vi "Delete_Unprocessed_Subtracks-1.vi"(4 "error IN":errorcluster, 5 "[IN] Before Pro\ncessing Tracks":T1(array[cluster]), 7 "[IN] Processed Tracks":T1(array[cluster])) -> (0 "error OUT":errorcluster, 1 "[OUT] Before Pro\ncessing Tracks":T1(array[cluster]), 3 "[IN] Filtered Tracks":T1(array[cluster]))   [LabVIEW 2013]
doc: "The subVI deletes the unprocessed points and tracks"
panel:
  out "# of deleted subtracks":i32
  out "# of deleted track groups":i32
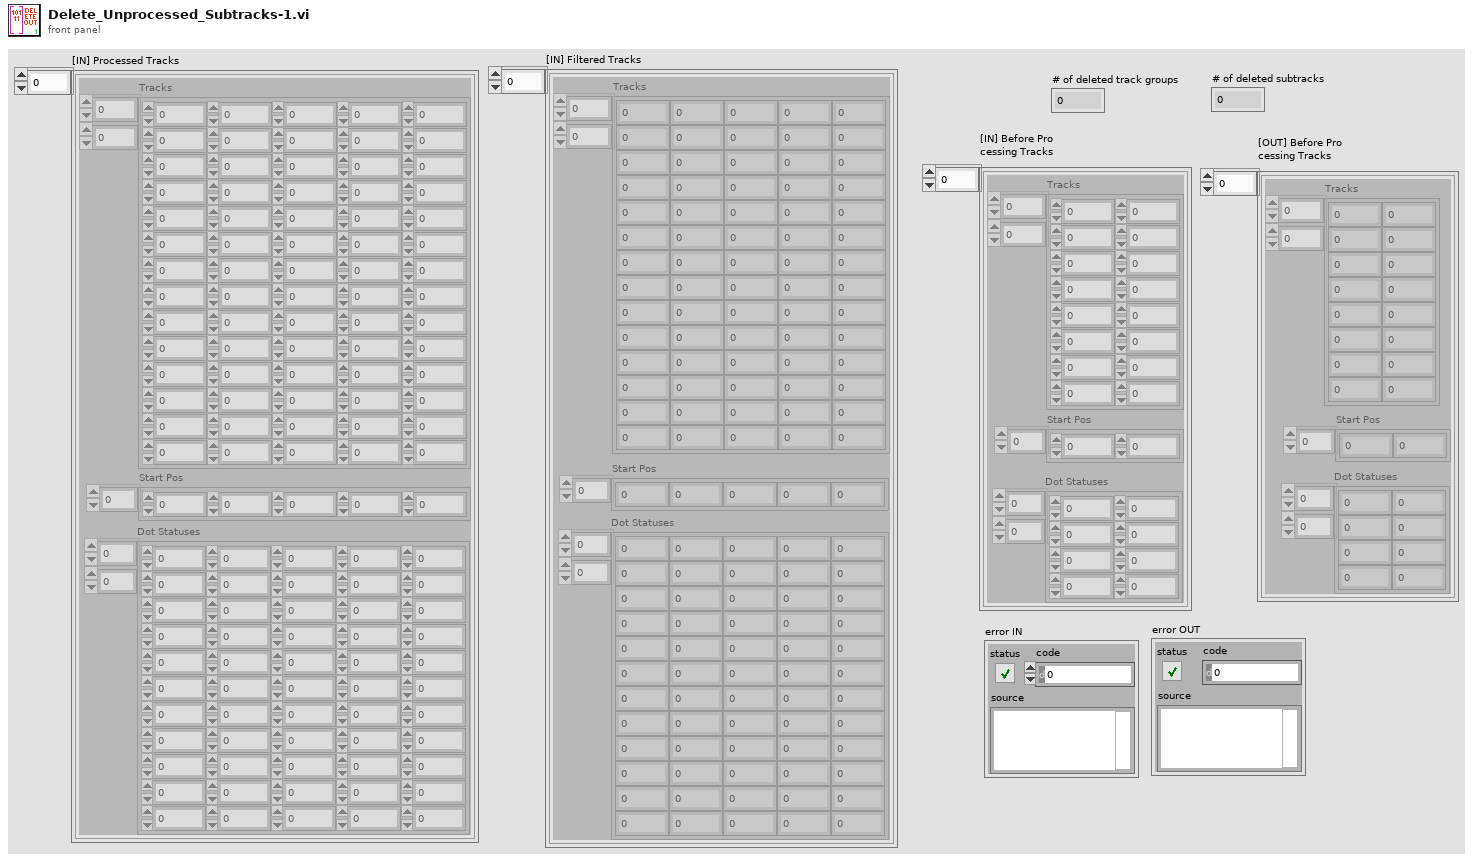
[diagram p1: front panel]
types:
  T1 = cluster{"Tracks":dbl[][], "Start Pos":i32[], "Dot Statuses":i16[][]}[]
  T2 = cluster{"Tracks":dbl[][], "Start Pos":i32[], "Dot Statuses":i16[][]}
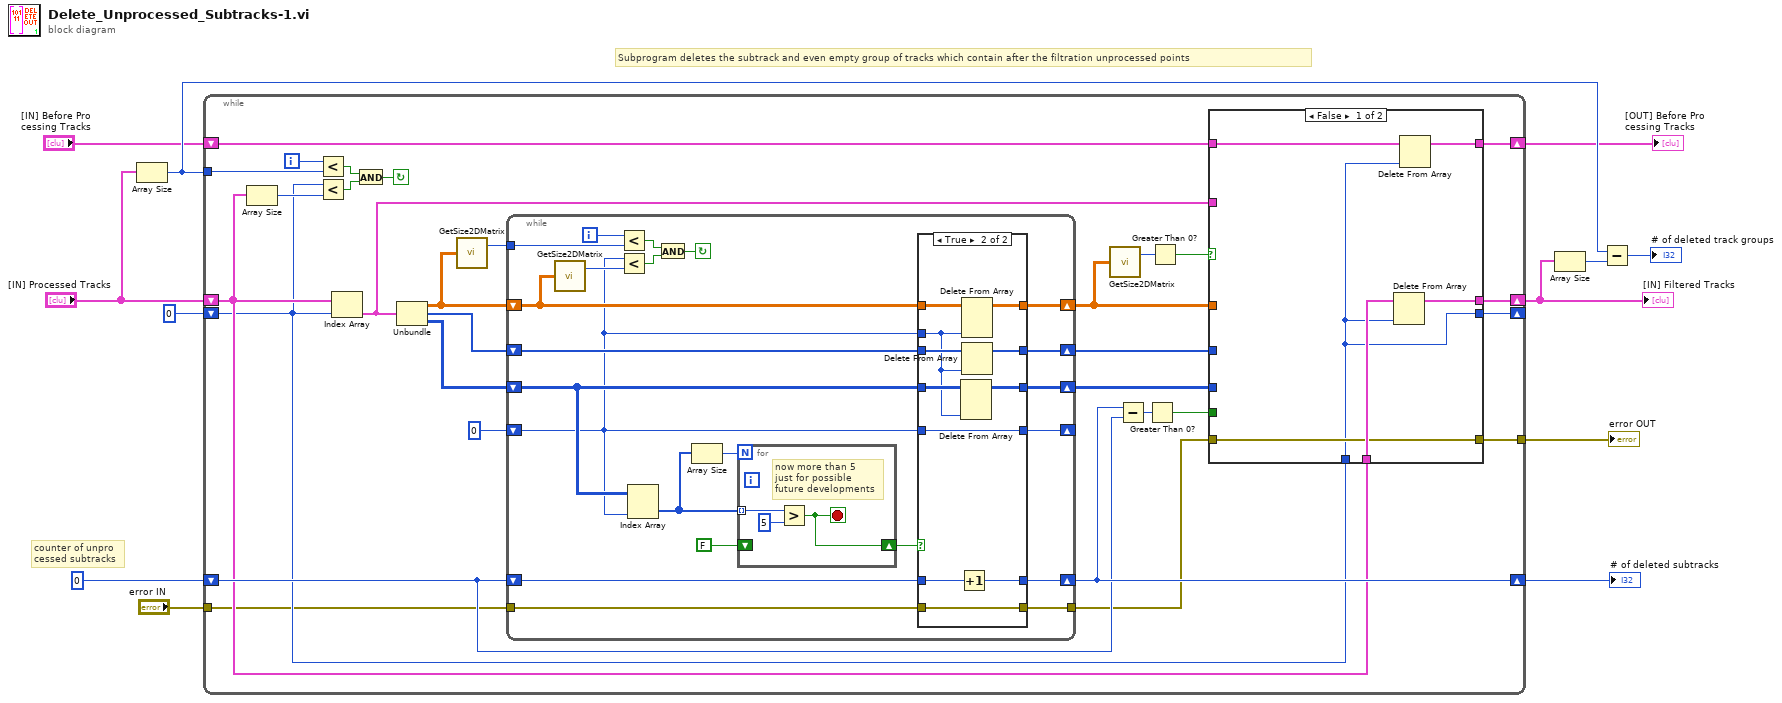
[diagram p0: block diagram]
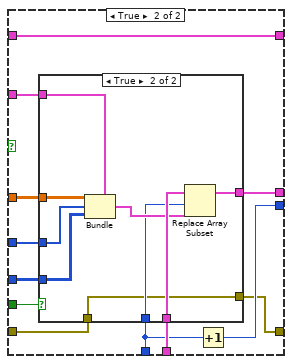
[diagram p2: hidden frame]
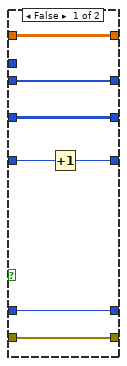
[diagram p4: hidden frame]
diagram:
  # "Subprogram deletes the subtrack and even empty group of tracks which contain after the filtration unprocessed points"
  # "counter of unpro\ncessed subtracks"
  n1 = Array Size(array="[IN] Processed Tracks") -> (size(s)=w7:i32)
  n2 = while {
    shift-right: [w19] -> w9
    shift-left: "[IN] Processed Tracks" -> [w21]
    shift-right: [w28] -> w3
    shift-left: 0 -> [w27]
    tunnel: w7 -> [w36]
    shift-right: [w18] -> _
    shift-left: 0 -> [w20]
    tunnel: "error IN" -> [w17]
    tunnel: [w15] -> w5
    shift-right: [w13] -> w1
    shift-left: "[IN] Before Pro\ncessing Tracks" -> [w14]
    i -> [w37]
    stop <- w30 continue-if-true
    n3 = Array Size(array=w21) -> (size(s)=w33:i32)
    n4 = Less?(x=w37, y=w36) -> (x < y?=w32:bool)
    n5 = Less?(x=w20, y=w33) -> (x < y?=w31:bool)
    n6 = Index Array(array=w21, index=w20) -> (element=w29:T2)
    n7 = And(x=w32, y=w31) -> (x .and. y?=w30:bool)
    n8 = Unbundle(w29) -> ("Tracks"=w41:dbl[][], "Start Pos"=w39:i32[], "Dot Statuses"=w42:i16[][])
    n9 = call "GetSize2DMatrix.vi"("Array IN (2D)"=w41) -> ("# Cols"=w40:i32)  [unwired: 1 out]
    n10 = while {
      shift-right: [w82] -> w24
      shift-left: w41 -> [w83]
      shift-right: [w78] -> w22
      shift-left: w42 -> [w79]
      tunnel: w40 -> [w92]
      shift-right: [w80] -> w23
      shift-left: w39 -> [w81]
      shift-right: [w76] -> _
      shift-left: 0 -> [w77]
      shift-right: [w74] -> w28
      shift-left: w27 -> [w75]
      tunnel: w17 -> [w73]
      tunnel: [w72] -> w16
      i -> [w85]
      stop <- w89 continue-if-true
      n11 = call "GetSize2DMatrix.vi"("Array IN (2D)"=w83) -> ("# Cols"=w93:i32)  [unwired: 1 out]
      n12 = Less?(x=w85, y=w92) -> (x < y?=w91:bool)
      n13 = Less?(x=w77, y=w93) -> (x < y?=w90:bool)
      n14 = Index Array(array=w79, index (col)=w77) -> (element=w87:i16[])  [unwired: 1 in]
      n15 = And(x=w91, y=w90) -> (x .and. y?=w89:bool)
      n16 = Array Size(array=w87) -> (size(s)=w88:i32)
      n17 = for {
        N: w88 -> [_]
        tunnel: w87 -> [w114] mode=indexing
        shift-right: [w112] -> w84
        shift-left: FALSE -> [_]
        stop <- w112 stop-if-true
        # "now more than 5\njust for possible \nfuture developments"
        n18 = Greater?(x=w114, y=i16 5) -> (0:w112:bool)
      }
      n19 = case shown="True" w84 {
        tunnel: w83 -> [w100 w111]
        tunnel: [w100 w110] -> w82
        tunnel: w77 -> [_ w106]
        tunnel: w81 -> [w99 w109]
        tunnel: [w99 w108] -> w80
        tunnel: w79 -> [w98 w107]
        tunnel: [w98 w105] -> w78
        tunnel: w77 -> [w97 w104]
        tunnel: [w96 w104] -> w76
        tunnel: w75 -> [w95 w103]
        tunnel: [w95 w102] -> w74
        tunnel: w73 -> [w94 w101]
        tunnel: [w94 w101] -> w72
        frame False {
          n20 = Increment(x=w97) -> (x+1=w96:i32)
        }
        frame True {
          n21 = Increment(x=w103) -> (x+1=w102:i32)
          n22 = Delete From Array(array=w107, index (col)=w106) -> (array with subset deleted=w105:i16[][])  [unwired: 2 in, 1 out]
          n23 = Delete From Array(array=w111, index (col)=w106) -> (array with subset deleted=w110:dbl[][])  [unwired: 2 in, 1 out]
          n24 = Delete From Array(array=w109, index=w106) -> (array with subset deleted=w108:i32[])  [unwired: 1 in, 1 out]
        }
      }
    }
    n25 = call "GetSize2DMatrix.vi"("Array IN (2D)"=w24) -> ("# Cols"=w35:i32)  [unwired: 1 out]
    n26 = Subtract(x=w28, y=w27) -> (x-y=w26:i32)
    n27 = Greater Than 0?(x=w26) -> (x > 0?=w25:bool)
    n28 = Greater Than 0?(x=w35) -> (x > 0?=w34:bool)
    n29 = case shown="False" w34 {
      tunnel: w29 -> [_ w59]
      tunnel: w25 -> [_ w60]
      tunnel: w24 -> [_ w58]
      tunnel: w23 -> [_ w57]
      tunnel: w22 -> [_ w56]
      tunnel: w21 -> [w48 w55]
      tunnel: w20 -> [w44 w53]
      tunnel: [w47 w54] -> w19
      tunnel: [w44 w52] -> w18
      tunnel: w16 -> [w46 w51]
      tunnel: [w46 w50] -> w15
      tunnel: w14 -> [w45 w49]
      tunnel: [w43 w49] -> w13
      frame False {
        n30 = Delete From Array(array=w48, index=w44) -> (array with subset deleted=w47:T1)  [unwired: 1 in, 1 out]
        n31 = Delete From Array(array=w45, index=w44) -> (array with subset deleted=w43:T1)  [unwired: 1 in, 1 out]
      }
      frame True {
        n32 = case shown="True" w60 {
          tunnel: w59 -> [_ w71]
          tunnel: w58 -> [_ w70]
          tunnel: w57 -> [_ w69]
          tunnel: w56 -> [_ w68]
          tunnel: w55 -> [w62 w67]
          tunnel: w53 -> [_ w64]
          tunnel: [w62 w65] -> w54
          tunnel: [w61 w63] -> w50
          tunnel: w51 -> [w61 w63]
          frame False {
          }
          frame True {
            n33 = Bundle(cluster=w71, "Tracks"=w70, "Start Pos"=w69, "Dot Statuses"=w68) -> (w66:T2)
            n34 = Replace Array Subset(array=w67, new element=w66, index=w64) -> (w65:T1)
          }
        }
        n35 = Increment(x=w53) -> (x+1=w52:i32)
      }
    }
  }
  "error OUT" <- w5
  "[IN] Filtered Tracks" <- w9
  "# of deleted subtracks" <- w3
  "[OUT] Before Pro\ncessing Tracks" <- w1
  n36 = Array Size(array=w9) -> (size(s)=w8:i32)
  n37 = Subtract(x=w7, y=w8) -> (x-y=→"# of deleted track groups":i32)
